vi "Autonomous_Independent.vi"() -> ()   [LabVIEW 2018]
doc: "This VI is called when autonomous begins, and will automatically be terminated when autonomous ends. You can carry out timed or sensor driven robot movement independently without needing to return to the caller."
uses:
  <vilib>/Rock Robotics/WPI/DriverStation/WPI_DriverStationDerivedRobotMode.ctl
  Global_Variables/Dashboard_Globals.vi
  <vilib>/Rock Robotics/Network Tables/NT Write String.vi
  Global_Variables/Refnum_Names.vi
  Global_Variables/Autonomous_Globals.vi
panel:
  out "Visited_Disabled":bool
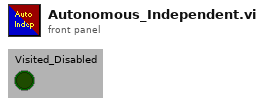
[diagram p1: front panel]
types:
  T1 = typedef "WPI_DriverStationDerivedRobotMode.ctl" = enum16{"Init", "Execute", "Stop"}
  T2 = typedef "Joystick_Controls.ctl" = cluster{"Pilot Left Joystick X":dbl, "Pilot Left Joystick Y":dbl, "Pilot A Button":bool, "Pilot B Button":bool, "Pilot X Button":bool, "Pilot Y Button":bool, "Pilot Left Bumper":bool, "Pilot Right Bumper":bool, "Pilot View Button":bool, "Pilot Menu Button":bool, "Pilot Left Joystick Press":bool, "Pilot Right Joystick Press":bool, "Pilot Left Trigger":dbl, "Pilot Right Joystick X":dbl, "Pilot Right Joystick Y":dbl, "Pilot Right Trigger":dbl, "Copilot Left Joystick X":dbl, "Copilot Left Joystick Y":dbl, "Copilot A Button":bool, "Copilot B Button":bool, "Copilot X Button":bool, "Copilot Y Button":bool, "Copilot Left Bumper":bool, "Copilot Right Bumper":bool, "Copilot View Button":bool, "Copilot Menu Button":bool, "Copilot Left Joystick Press":bool, "Copilot Right Joystick Press":bool, "Copilot Left Trigger":dbl, "Copilot Right Joystick X":dbl, "Copilot Right Joystick Y":dbl, "Copilot Right Trigger":dbl, "Pilot D-pad North":bool, "Pilot D-pad South":bool, "Pilot D-pad East":bool, "Pilot D-pad West":bool, "Pilot D-pad NE ":bool, "Pilot D-pad SE":bool, "Pilot D-pad SW":bool, "Pilot D-pad NW":bool, "CoPilot D-pad North":bool, "CoPilot D-pad South":bool, "CoPilot D-pad East":bool, "CoPilot D-pad West":bool, "CoPilot D-pad NE":bool, "CoPilot D-pad SE":bool, "CoPilot D-pad SW":bool, "CoPilot D-pad NW":bool, "Pilot Left Trigger Pressed":bool, "Pilot Right Trigger Pressed":bool, "CoPilot Left Trigger Pressed":bool, "CoPilot Right Trigger Pressed":bool}
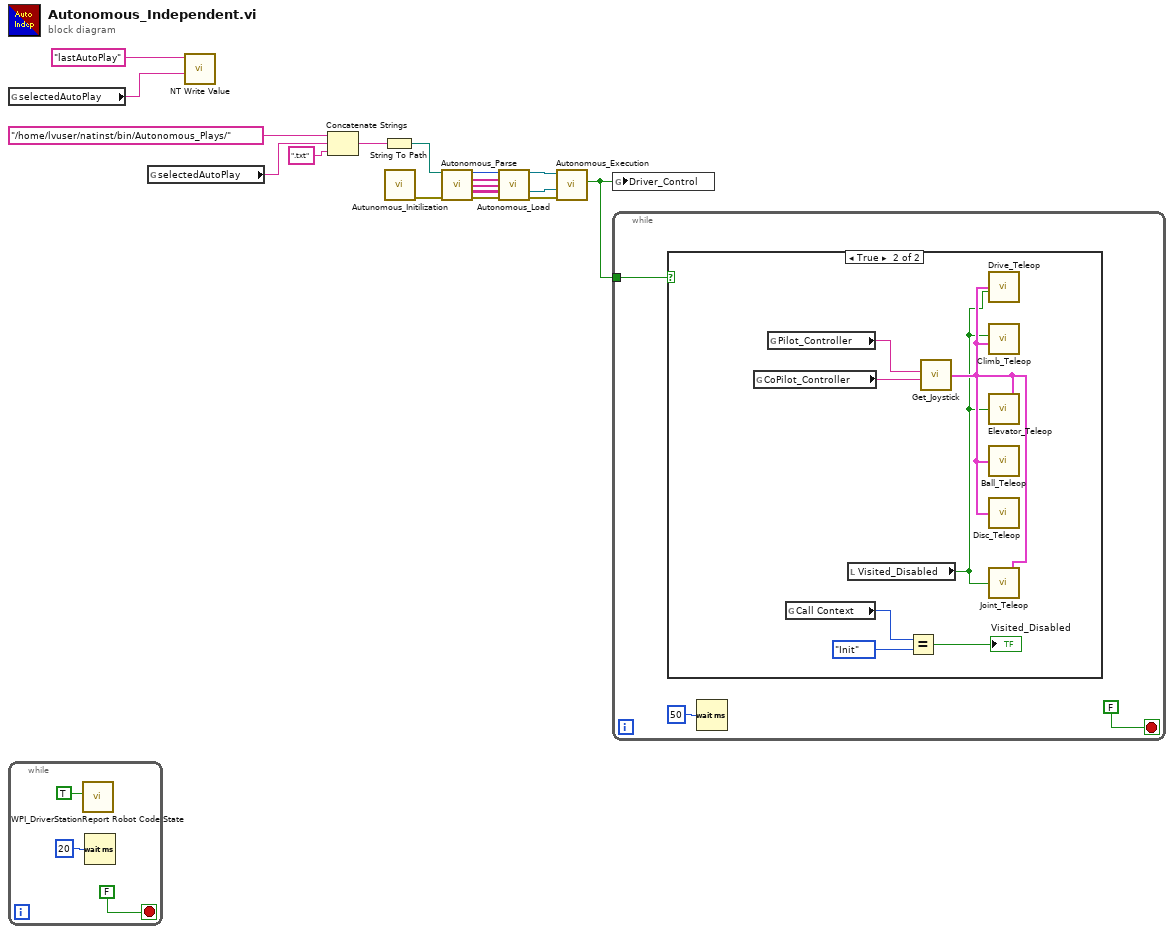
[diagram p0: block diagram]
diagram:
  n1 = global read "Dashboard_Globals.vi" "selectedAutoPlay"() -> (w16:string)
  n2 = while {
    stop <- FALSE stop-if-true
    n3 = call <vilib>:"WPI_DriverStationReport Robot Code State.vi"("Autonomous"=TRUE) -> ()  [unwired: 10 in, 1 out]
    n4 = Wait (ms)(milliseconds to wait=u32 20) -> ()  [unwired: 1 out]
  }
  n5 = global read "Dashboard_Globals.vi" "selectedAutoPlay"() -> (w12:string)
  n6 = call-poly <vilib>:"NT Write Value.vi"("String"=w16, "Name"="lastAutoPlay") -> ()  [unwired: 9 in, 1 out]
  n7 = Concatenate Strings("/home/lvuser/natinst/bin/Autonomous_Plays/" ("string"), w12, ".txt" ("string")) -> (w10:string)
  n8 = String To Path(string=w10) -> (path=w11:path)
  n9 = call "Autunomous_Initilization.vi"() -> ("errror out"=w15:errorcluster)  [unwired: 11 in]
  n10 = call "Autonomous_Parse.vi"("File Path"=w11, "error in"=w15) -> ("Number of Commands"=w9:i32, "Subsystems"=w8:string[], "Commands"=w6:string[], "Inputs"=w5:string[][], "errror out"=w7:errorcluster)  [unwired: 7 in, 2 out]
  n11 = call "Autonomous_Load.vi"("Number of Commands"=w9, "Subsystems"=w8, "Commands"=w6, "Inputs"=w5, "error in"=w7) -> ("Queue_Key"=w3:refnum<queue>, "Autonomous_Queue"=w2:refnum<queue>, "errror out"=w4:errorcluster)  [unwired: 8 in]
  n12 = call "Autonomous_Execution.vi"("error in"=w4, "Autonomous_Queue"=w2, "Queue Key"=w3) -> ("Done"=w1:bool)  [unwired: 8 in]
  n13 = global write "Autonomous_Globals.vi" "Driver_Control"(w1) -> ()
  n14 = while {
    tunnel: w1 -> [w23]
    stop <- FALSE stop-if-true
    n15 = case shown="True" w23 {
      frame False {
      }
      frame True {
        n16 = global read "Refnum_Names.vi" "CoPilot_Controller"() -> (w30:string)
        n17 = global read "Refnum_Names.vi" "Pilot_Controller"() -> (w28:string)
        n18 = global read "Autonomous_Globals.vi" "Call Context"() -> (w26:T1)
        n19 = local read "Visited_Disabled"() -> (w24:bool)
        n20 = Equal?(x=w26, y=WPI_DriverStationDerivedRobotMode."Init") -> (x = y?=→"Visited_Disabled":bool)
        n21 = call "Get_Joystick.vi"("Joystick_One"=w28, "Joystick_Two"=w30) -> ("Joystick_Out"=w29:T2)  [unwired: 5 in]
        n22 = call "Drive_Teleop.vi"("Joystick_Out"=w29, "Visited_Disabled"=w24) -> ()  [unwired: 3 in]
        n23 = call "Climb_Teleop.vi"("Joystick_Out"=w29, "Visited_Disabled"=w24) -> ()  [unwired: 3 in]
        n24 = call "Elevator_Teleop.vi"("Joystick_Out"=w29, "Visited_Disabled"=w24) -> ()
        n25 = call "Ball_Teleop.vi"("Joystick_Out"=w29) -> ()  [unwired: 1 in]
        n26 = call "Disc_Teleop.vi"("Joystick_Out"=w29) -> ()  [unwired: 1 in]
        n27 = call "Joint_Teleop.vi"("Joystick_Out"=w29, "Visited_Disabled"=w24) -> ()
      }
    }
    n28 = Wait (ms)(milliseconds to wait=u32 50) -> ()  [unwired: 1 out]
  }
